vi "Demo_Grab+.vi"() -> ()   [LabVIEW 2024]
doc: "Grab any video source supported by QuickTime (internal, USB, FW, etc).\nThe output image can be compressed with any QT supported format (See image->compressed_data).\nSet Dialogs to 1 in Frame grabber settings to use the standard QT dialog.\n\nChris Salzmann © 1994-2003"
uses:
  <userlib>/ImageProcessing/QTLIB_2595_LV86/QT_Private.ctl
  <userlib>/ImageProcessing/QTLIB_2595_LV86/QT_Video.ctl
  <userlib>/ImageProcessing/QTLIB_2595_LV86/QT_Compression.ctl
  <userlib>/ImageProcessing/QTLIB_2595_LV86/QT_Thresholds.ctl
  <userlib>/ImageProcessing/QTLIB_2595_LV86/QT_FrameGrabber.ctl
panel:
  in  "Case Constant\n(See Context Help)":bool=TRUE
  in  "Color Box 3":u32(colorbox)=255
  in  "Color Box 2":u32(colorbox)=65280
  in  "Color Box":u32(colorbox)=16711680
  out "B":picture
  out "G":picture
  out "R":picture
  in  "Blue":i32(slide)=242 scale=0.0..255.0
  in  "Green":i32(slide)=182 scale=0.0..255.0
  in  "Red":i32(slide)=219 scale=0.0..255.0
  out "Picture B&W/Alpha channel":picture
  in  "BW":i32(slide)=217 scale=0.0..255.0
  in  "Compression":i32(slide)=745 scale=0.0..1024.0 scale format="%x"
  in  "Codec (raw )":T1(ring)=enum."jpeg"
  out "error out":errorcluster
  in  "White l.":dbl(slide)=80.61224489795919 scale=0.0..100.0
  in  "Black l.":dbl(slide)=14.285714285714286 scale=0.0..100.0
  in  "Sharp":dbl(slide)=1.7857142857142858 scale=0.0..100.0
  in  "Contr":dbl(slide)=67.85714285714286 scale=0.0..100.0
  in  "Bright":dbl(slide)=10.714285714285715 scale=0.0..100.0
  in  "Sat":dbl(slide)=83.92857142857143 scale=0.0..100.0
  in  "Hue":dbl(slide)=50.0 scale=0.0..100.0
  out "CIN info":string="© Chris 94-2005, QT Fat-CIN, rev: 2583, FATQTCin.c, Jul 28 2005, 18:12:54"
  out "QT Version":string="QuickTime v. 652 "
  out "Picture":picture
  in  "stop":bool
  in  "Frame Grabber Settings":T2={"Name"="", "Digitizer"=2, "Input"=1, "Width"=160, "Height"=120, "Input format"=enum."NTSC", "Frame rate"=0.0, "Reserved"=0, "Dialogs"=0} {"Frame rate" format="%#1_6g"; "Dialogs" format="%.0b"}
  # "Grab any video source supported by QuickTime (internal, USB, FW, etc).\nThe output image can be compressed with any QT supported format (See image->compressed_data).\nSet Dialogs to 1 in Frame grabber settings to use the standard QT dialog.\n\nChris Salzmann © 1994-2005"
  # "No compression\n-> raw"
  # "Test pattern"
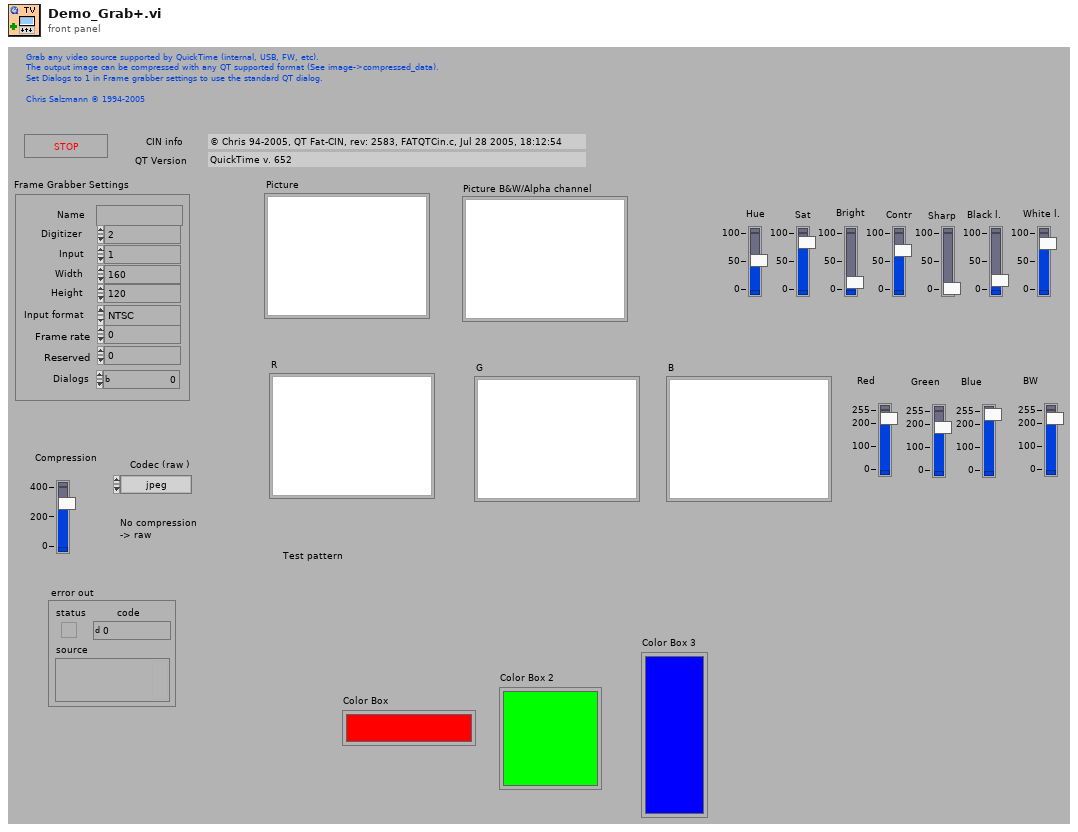
[diagram p1: front panel]
types:
  T1 = enum16{"rle ", "WRLE", "cvid", "yuv2", "dvcp", "dvc ", "dvpp", "smc ", "h261", "h263", "mjp2", "mjpa", "mjpb", "mp4v", "raw ", "VP31", "jpeg", "8BPS", "png ", "SVQ1", "SVQ3", "tga ", "tiff", "rpza", "ZyGo"}
  T2 = typedef "QT_FrameGrabber.ctl" = cluster{"Name":string, "Digitizer":i32, "Input":i32, "Width":i32, "Height":i32, "Input format":enum32{"NTSC", "PAL", "Secam"}, "Frame rate":dbl, "Reserved":i32, "Dialogs":u32}
  T3 = typedef "QT_Thresholds.ctl" = cluster{"BW threshold":dbl, "Red threshold":dbl, "Green threshold":dbl, "Blue threshold":dbl, "Crop rgn":cluster{"left":i16, "top":i16, "right":i16, "bottom":i16}, "Reserved":i32}
  T4 = typedef "QT_Compression.ctl" = cluster{"Compression":i32, "Format":i32, "Codec":i32, "Comp. Quality":i32, "Key Frame":i32, "Dialogs":u32}
  T5 = typedef "QT_Video.ctl" = cluster{"Color format":u32, "Hue":dbl, "Saturation":dbl, "Brightness":dbl, "Contrast":dbl, "Sharpness":dbl, "Black Level":dbl, "White Level":dbl, "Options":i32, "Dialogs":u32}
  T6 = typedef "QT_Private.ctl" = cluster{"reserved 1":i32, "reserved 2":i32, "reserved 3":i32, "reserved 4":i32}
  T7 = typedef "QT_Ref.ctl" = refnum<k1>
  T8 = typedef "QT_Image.ctl" = cluster{"Width":i32, "Height":i32, "Depth":i32, "data":u8[], "Compressed data":u8[], "Color table":u32[], "Duration":i32, "Options":i32, "Timestamp":i32, "ID":i32, "Reserved":i32, "Dialogs":u32}
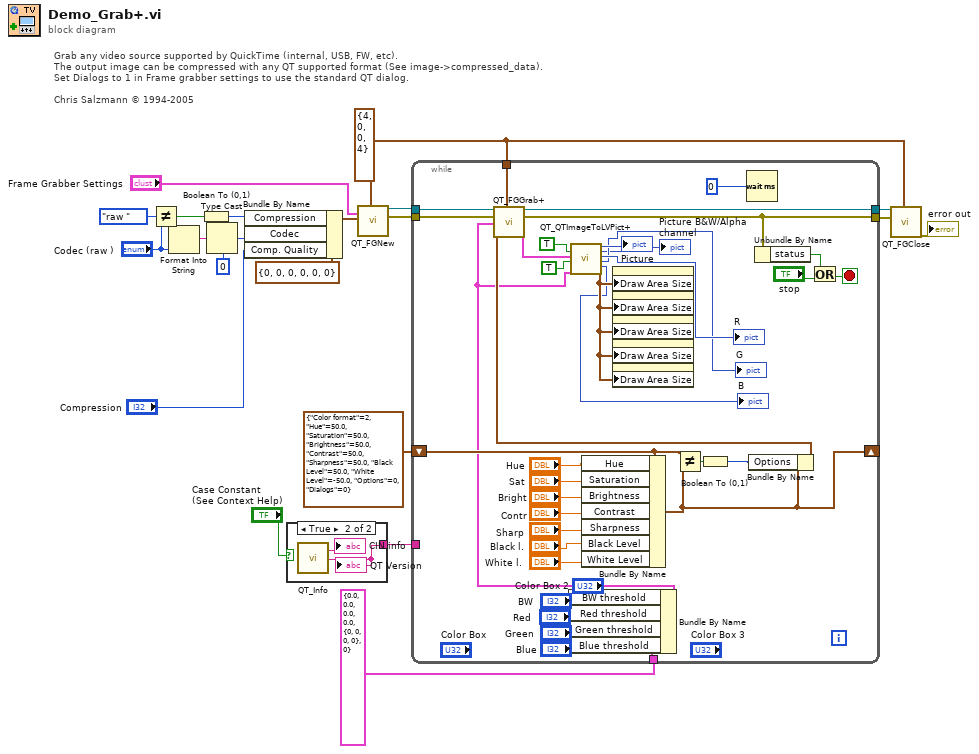
[diagram p0: block diagram]
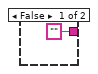
[diagram p2: hidden frame]
diagram:
  w7 = T6 {"reserved 1"=4, "reserved 2"=0, "reserved 3"=0, "reserved 4"=4} ("Private")
  # "Grab any video source supported by QuickTime (internal, USB, FW, etc).\nThe output image can be compressed with any QT supported format (See image->compressed_data).\nSet Dialogs to 1 in Frame grabber settings to use the standard QT dialog.\n\nChris Salzmann © 1994-2005"
  n1 = Not Equal?(x=T1."raw " ("codec (raw )"), y="Codec (raw )") -> (x != y?=w3:bool)
  n2 = Format Into String("Codec (raw )") -> (resulting string=w12:string)  [unwired: 3 in, 1 out]
  n3 = Boolean To (0,1)(Boolean=w3) -> (0, 1=w2:i16)
  n4 = Type Cast(type=0 ("Codec"), x=w12) -> (*(type *) &x=w11:i32)
  n5 = Bundle By Name(cluster=T4 {"Compression"=0, "Format"=0, "Codec"=0, "Comp. Quality"=0, "Key Frame"=0, "Dialogs"=0} ("Compression Settings"), "Compression"=w2, "Codec"=w11, "Comp. Quality"="Compression") -> (w13:T4)
  n6 = case shown="True" "Case Constant\n(See Context Help)" {
    tunnel: ["" ("QT Version") w24] -> w6
    frame False {
    }
    frame True {
      n7 = call <userlib>:"QT_Info.vi"() -> ("CIN info"=→"CIN info":string, "QT Version"=w24:string)  [unwired: 3 in, 15 out]
      "QT Version" <- w24
    }
  }
  n8 = call <userlib>:"QT_FGNew.vi"("Frame Grabber Settings"="Frame Grabber Settings", "Compression Settings"=w13, "Private"=w7) -> ("QT Ref Out"=w20:T7, "error out"=w15:errorcluster)  [unwired: 2 in, 13 out]
  n9 = while {
    shift-left: T5 {"Color format"=2, "Hue"=50.0, "Saturation"=50.0, "Brightness"=50.0, "Contrast"=50.0, "Sharpness"=50.0, "Black Level"=50.0, "White Level"=-50.0, "Options"=0, "Dialogs"=0} ("Video Settings") -> [w44]
    shift-right: [w42] -> _
    tunnel: [w55] -> w18
    tunnel: w15 -> [w56]
    tunnel: w7 -> [w57]
    tunnel: [w59] -> w21
    tunnel: w20 -> [w60]
    tunnel: w6 -> [_]
    tunnel: T3 {"BW threshold"=0.0, "Red threshold"=0.0, "Green threshold"=0.0, "Blue threshold"=0.0, "Crop rgn"={"left"=0, "top"=0, "right"=0, "bottom"=0}, "Reserved"=0} ("Thresholds") -> [w36]
    stop <- w54 stop-if-true
    n10 = Bundle By Name(cluster=w36, "BW threshold"="BW", "Red threshold"="Red", "Green threshold"="Green", "Blue threshold"="Blue") -> (w30:T3)
    n11 = Bundle By Name(cluster=w44, "Hue"="Hue", "Saturation"="Sat", "Brightness"="Bright", "Contrast"="Contr", "Sharpness"="Sharp", "Black Level"="Black l.", "White Level"="White l.") -> (w42:T5)
    n12 = Not Equal?(x=w44, y=w42) -> (x != y?=w43:bool)
    n13 = Boolean To (0,1)(Boolean=w43) -> (0, 1=w37:i16)
    n14 = Wait (ms)(milliseconds to wait=u32 0) -> ()  [unwired: 1 out]
    n15 = Bundle By Name(cluster=w42, "Options"=w37) -> (w41:T5)
    n16 = call <userlib>:"QT_FGGrab+.vi"("QT Ref In"=w60, "Video Settings in"=w41, "error in (no error)"=w56, "Thresholds"=w30, "Private"=w57) -> ("QT Ref Out"=w59:T7, "Image/Movie Out"=w40:T8, "error out"=w55:errorcluster)  [unwired: 2 in, 10 out]
    n17 = call <userlib>:"QT_QTImageToLVPict+.vi"("Draw info"=TRUE, "Image/Movie Out"=w40, "BW image"=TRUE, "Thresholds"=w30) -> ("Picture color"=→"Picture":picture, "Picture B&W/Alpha channel"=→"Picture B&W/Alpha channel":picture, "R"=→"R":picture, "G"=→"G":picture, "B"=→"B":picture, "Pict Draw Area Size"=w29:cluster{"Width":i16, "Height":i16})  [unwired: 10 out]
    n18 = property on="Picture" class="Pict"("Draw Area Size"=w29) -> ()  [unwired: 2 in, 2 out]
    n19 = property on="Picture B&W/Alpha channel" class="Pict"("Draw Area Size"=w29) -> ()  [unwired: 2 in, 2 out]
    n20 = property on="R" class="Pict"("Draw Area Size"=w29) -> ()  [unwired: 2 in, 2 out]
    n21 = property on="G" class="Pict"("Draw Area Size"=w29) -> ()  [unwired: 2 in, 2 out]
    n22 = property on="B" class="Pict"("Draw Area Size"=w29) -> ()  [unwired: 2 in, 2 out]
    n23 = Unbundle By Name(w55) -> ("status"=w52:bool)
    n24 = Or(x=w52, y="stop") -> (x .or. y?=w54:bool)
  }
  n25 = call <userlib>:"QT_FGClose.vi"("QT Ref In"=w21, "error in (no error)"=w18, "Private"=w7) -> ("error out"=→"error out":errorcluster)  [unwired: 1 in, 15 out]
